vi "PRL Signal Calculator.vi"(0 "Phasor Values In":csg[][](array[numeric]), 1 "Cut Index":i32, 5 "Analog Values In":sgl[][](array[numeric]), 7 "Digital Values In":bool[][](array[boolean])) -> (12 "Signal Names In":T1)   [LabVIEW 2018, in "S3DK.lvlib" / "PMU Recorder Light.lvlib"]
uses:
  PMU Recorder Light.lvlib
panel:
  out "Signal Names Test":T1={"Phasor"=["Hasle/Halden-U", "Hasle/Borgvik-U", "Hasle/Borgvik-I", "Hasle/Halden-I", "Hasle/Roed-I", "Hasle/Tegneby-I", "NedreRossaga/Rana-U", "NedreRossaga/Rana-I", "Ben 667/420:Ba1:U_L1", "Ben 667/420:Ba1:U_L2", "Ben 667/420:Ba1:U_L3", "Ben 667/420:Ba1:I_L1", "Ben 667/420:Ba1:I_L2", "Ben 667/420:Ba1:I_L3", "Ben 667/420:Of1:U_L1", "Ben 667/420:Of1:U_L2", "Ben 667/420:Of1:U_L3", "Ben 667/420:Of1:I_L1", "Ben 667/420:Of1:I_L2", "Ben 667/420:Of1:I_L3", "Keminmaa/PK1", "Keminmaa/PK2", "Keminmaa/SELLEE 1.1/2", "Keminmaa/SB 1.7/8", "Keminmaa/PR 1.9/10", "Keminmaa/PT 1.11/12", "PETAJASKOSKI/V1LPM", "PETAJASKOSKI/I1WPM", "PETAJASKOSKI/I1XPM"], "Analog"=["Hasle/frequency", "Hasle/frequency-delta", "NedreRossaga/frequency", "NedreRossaga/frequency-delta", "Ben 667/frequency", "Ben 667/frequency-delta", "Keminmaa/frequency", "Keminmaa/frequency-delta", "PETAJASKOSKI/frequency", "PETAJASKOSKI/frequency-delta"], "Digital"=[]}
  in  "Digital":i32[](listbox)
  in  "Analog":i32[](listbox)
  in  "Phasor":i32[](listbox)
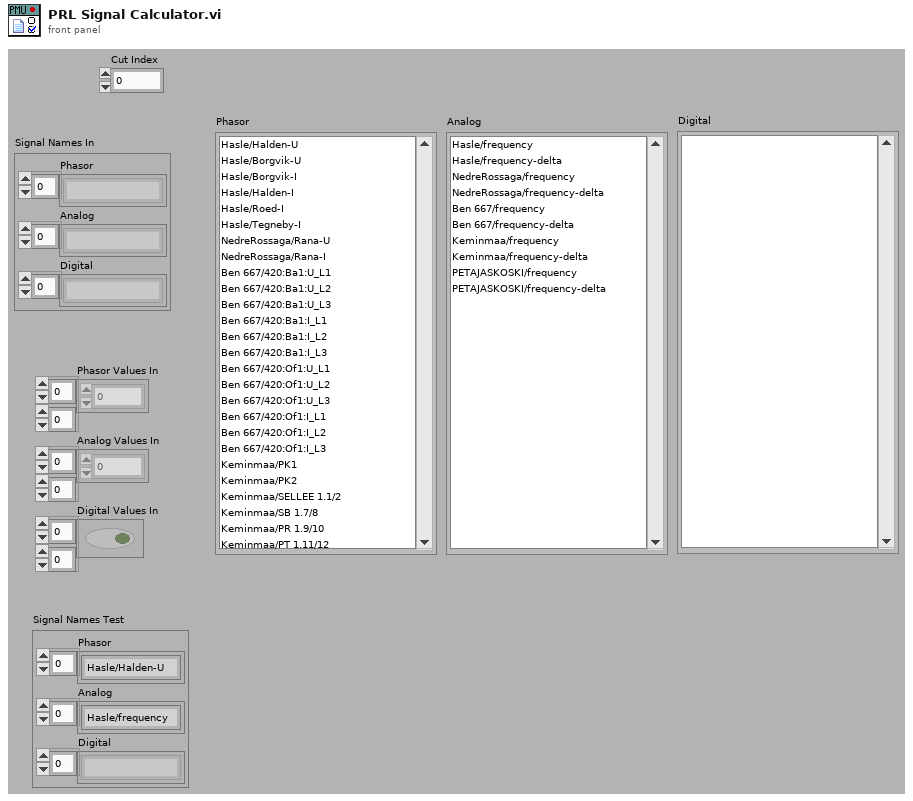
[diagram p1: front panel]
types:
  T1 = cluster{"Phasor":string[], "Analog":string[], "Digital":string[]}
  T2 = cluster{"Item Names":string[], "Item Names":string[], "Item Names":string[]}
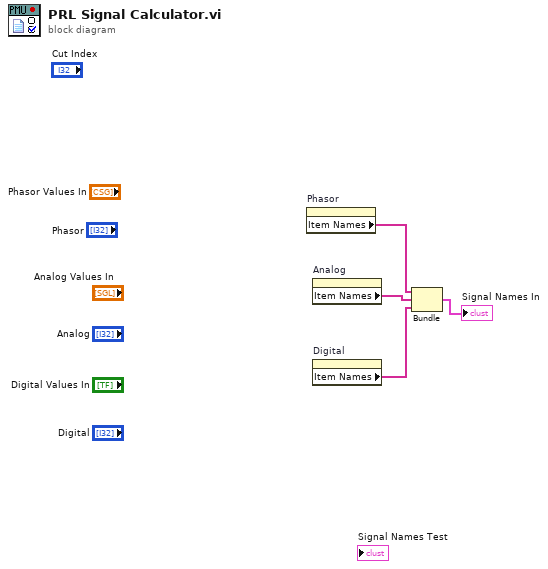
[diagram p0: block diagram]
diagram:
  n1 = property on="Phasor" class="LstBox (strict)"() -> ("Item Names"=w4:string[])  [unwired: 2 in, 2 out]
  n2 = property on="Analog" class="LstBox (strict)"() -> ("Item Names"=w3:string[])  [unwired: 2 in, 2 out]
  n3 = property on="Digital" class="LstBox (strict)"() -> ("Item Names"=w2:string[])  [unwired: 2 in, 2 out]
  n4 = Bundle("Item Names"=w4, "Item Names"=w3, "Item Names"=w2) -> (→"Signal Names In":T2)  [unwired: 1 in]
